vi "test_Create FPGA Addon_Group Scalars.vi"(8 "error in (no error)":errorcluster, 11 "TestCase in":refnum<class "FPGA Addon Scripting API Unit Tests.lvclass">=refnum) -> (0 "error out":errorcluster, 3 "TestCase out":refnum<class "FPGA Addon Scripting API Unit Tests.lvclass">)   [LabVIEW 2026, in "FPGA Addon Scripting API Unit Tests.lvclass"]
uses:
  FPGA Addon Scripting API Unit Tests.lvclass
  FPGA Addon Test Class/FPGA Addon Test Class.lvclass
  APIs/Scripting API/Scripting API.lvlib
  Addon/Addon Shared/FPGA Addon Shared.lvlib
  Addon/Addon Shared/Types/FG Action.ctl
  <vilib>/NI VeriStand/Custom Device Tools/Custom Device Utility Library/Custom Device Utility Library.lvlib
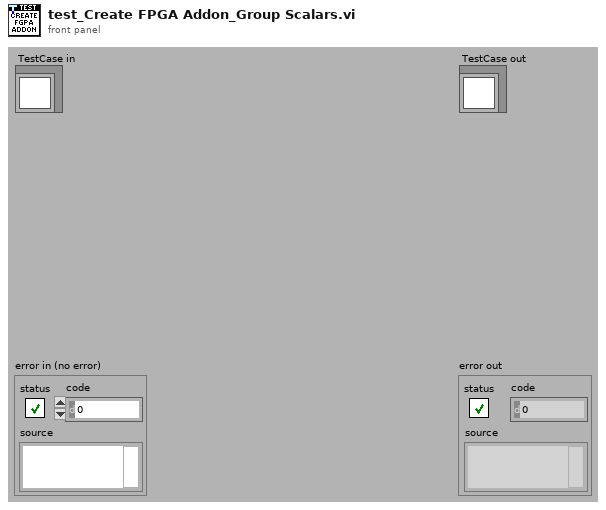
[diagram p1: front panel]
types:
  T1 = typedef "FPGA Addon Shared.lvlib/FG Action.ctl" = enum8{"GET", "SET"}
  T2 = typedef "Custom Device API.lvlib/Custom Device Item Ref.ctl" = u64
  T3 = typedef "FPGA Addon Shared.lvlib/FPGA Settings.ctl" = cluster{"Bitfile path":path, "RIO Device Address":string, "Group":bool}
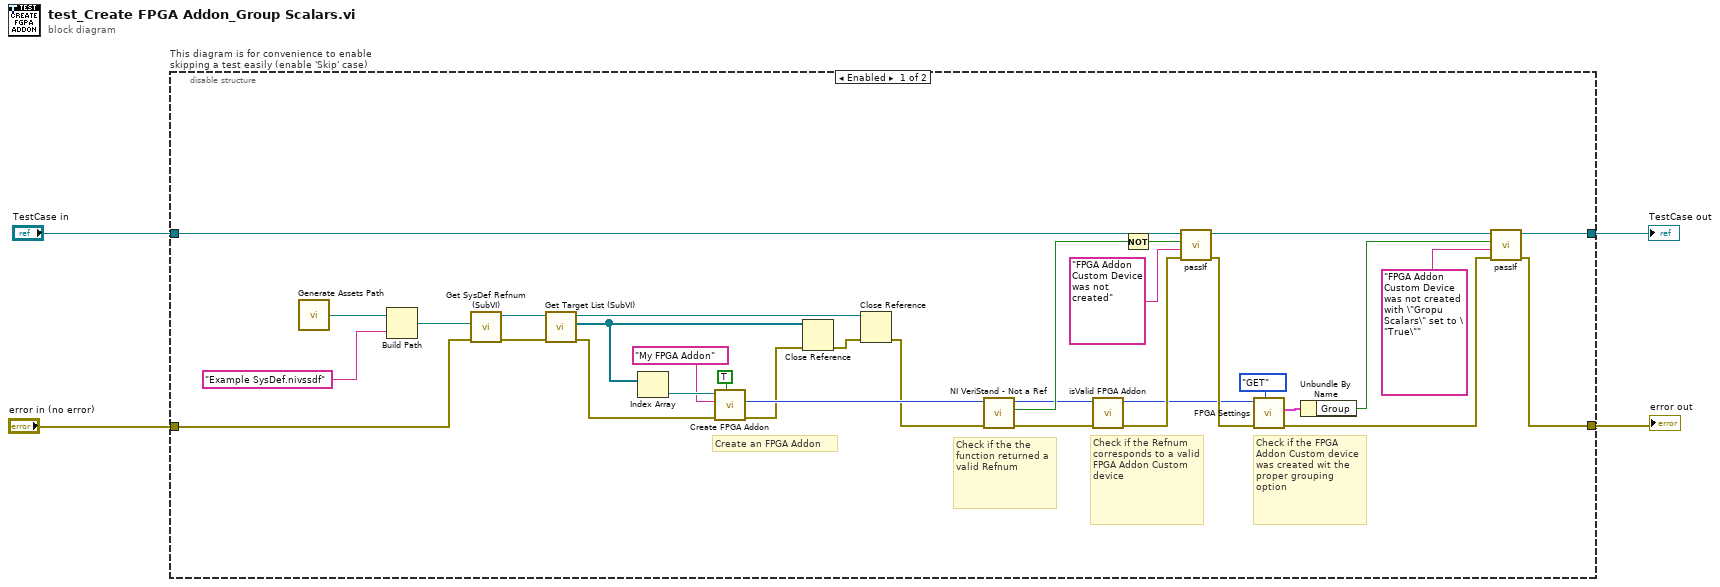
[diagram p0: block diagram]
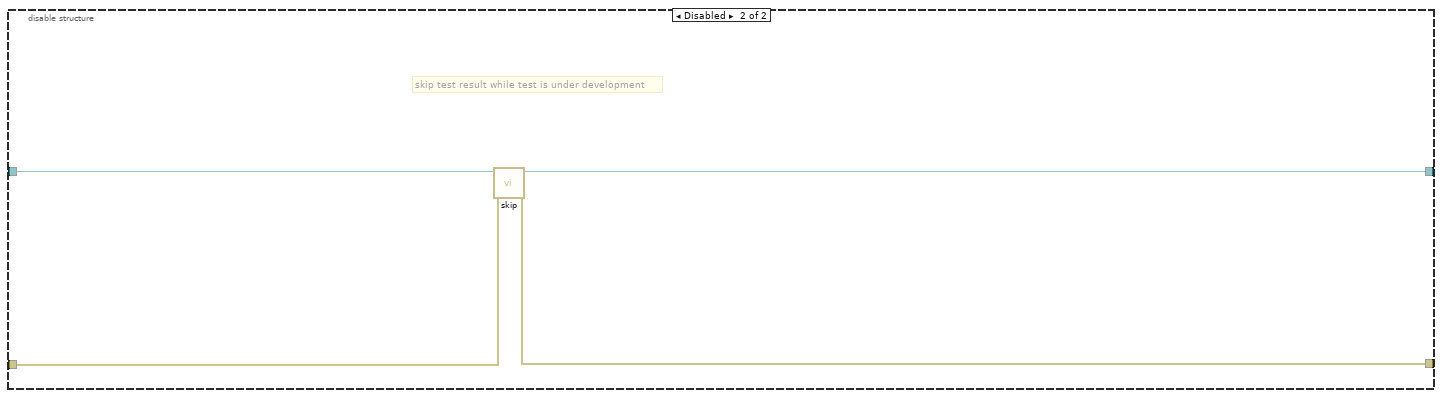
[diagram p2: hidden frame]
diagram:
  n1 = disable-structure "This diagram is for convenience to enable skipping a test easily (enable 'Skip' case)" shown="Enabled" {
    disable-tunnel: "TestCase in" -> [w27 w41]
    disable-tunnel: [w17 w39] -> w1
    disable-tunnel: [w16 w40] -> w3
    disable-tunnel: "error in (no error)" -> [w31 w38]
    frame Enabled {
      # "Check if the FPGA Addon Custom device was created wit the proper grouping option"
      # "Check if the Refnum corresponds to a valid FPGA Addon Custom device"
      # "Check if the the function returned a valid Refnum"
      # "Create an FPGA Addon"
      n2 = call "Generate Assets Path.vi"() -> ("Assets path"=w37:path)
      n3 = Build Path(base path=w37, name or relative path="Example SysDef.nivssdf") -> (appended path=w35:path)
      n4 = call "Get SysDef Refnum (SubVI).vi"("error in (no error)"=w31, "System Definition path"=w35) -> ("error out"=w30:errorcluster, "NationalInstruments.VeriStand.SystemDefinitionAPI.SystemDefinition"=w34:refnum<k39>)  [unwired: 8 in]
      n5 = call "Get Target List (SubVI).vi"("error in (no error)"=w30, "NationalInstruments.VeriStand.SystemDefinitionAPI.SystemDefinition"=w34) -> ("error out"=w29:errorcluster, "Target List Refnums"=w15:refnum<k39>[], "NationalInstruments.VeriStand.SystemDefinitionAPI.SystemDefinition"=w14:refnum<k39>)  [unwired: 7 in]
      n6 = Index Array(array=w15) -> (element=w33:refnum<k39>)  [unwired: 1 in]
      n7 = call "Create FPGA Addon.vi"("group scalars"=TRUE, "error in"=w29, "FPGA addon name"="My FPGA Addon", "NationalInstruments.VeriStand.SystemDefinitionAPI.Target"=w33) -> ("error out"=w11:errorcluster, "FPGA addon refnum"=w26:T2)  [unwired: 5 in, 1 out]
      n8 = Close Reference(reference=w15, error in (no error)=w11) -> (error out=w13:errorcluster)
      n9 = Close Reference(reference=w14, error in (no error)=w13) -> (error out=w12:errorcluster)
      n10 = call <vilib>:"NI VeriStand - Not a Ref.vi"("error in (no error)"=w12, "Item Ref"=w26) -> ("error out"=w7:errorcluster, "Not a Ref"=w25:bool, "Item Ref out"=w8:T2)  [unwired: 7 in]
      n11 = call "isValid FPGA Addon.vi"("error in"=w7, "FPGA Addon refnum in"=w8) -> ("error out"=w6:errorcluster, "FPGA Addon refnum out"=w5:T2)  [unwired: 8 in]
      n12 = Not(x=w25) -> (.not. x?=w24:bool)
      n13 = call-dynamic "passIf.vi"("error in (no error)"=w6, "message (\"\")"="FPGA Addon Custom Device was not created" ("message (\"\")"), "pass"=w24, "TestCase in"=w27) -> ("error out"=w22:errorcluster, "TestCase out"=w20:refnum<class "FPGA Addon Scripting API Unit Tests.lvclass">)  [unwired: 6 in]
      n14 = call "FPGA Settings.vi"("Action"=FG_Action."GET", "error in (no error)"=w22, "Item Ref"=w5) -> ("error out"=w18:errorcluster, "FPGA Settings"=w21:T3)  [unwired: 6 in, 1 out]
      n15 = Unbundle By Name(w21) -> ("Group"=w10:bool)
      n16 = call-dynamic "passIf.vi"("error in (no error)"=w18, "message (\"\")"="FPGA Addon Custom Device was not created with \"Gropu Scalars\" set to \"True\"" ("message (\"\")"), "pass"=w10, "TestCase in"=w20) -> ("error out"=w16:errorcluster, "TestCase out"=w17:refnum<class "FPGA Addon Scripting API Unit Tests.lvclass">)  [unwired: 6 in]
    }
    frame Disabled {
      # "skip test result while test is under development"
      n17 = call <vilib>:"skip.vi"("error in (no error)"=w38, "TestCase in"=w41) -> ("error out"=w40:errorcluster, "TestCase out"=w39:refnum<class "FPGA Addon Scripting API Unit Tests.lvclass">)  [unwired: 8 in]
    }
  }
  "error out" <- w3
  "TestCase out" <- w1
